vi "Packet RX Only.vi"() -> ()   [LabVIEW 2017, in "My Network Host v1.lvlib"]
uses:
  My Network Host v1.lvlib
  <vilib>/userdefined/Silver/nirio_resource_slv.ctl
  <vilib>/rvi/interface/common/niFpgaWaitOnOcc.vi
  <vilib>/Utility/error.llb/Error Cluster From Error Code.vi
  <vilib>/rvi/errors/niLvFpgaAdjustHostInterfaceError.vi
  <vilib>/FPGAPlugInAG/Dynamic/niLvFpga_Close_Dynamic.vi
  <vilib>/rvi/interface/nirviMethod/nirviMethod.xnode
  <vilib>/rvi/interface/nirviReadWriteControl/nirviReadWriteControl.xnode
  <vilib>/rvi/interface/nirviCloseFPGA/nirviCloseFPGA.xnode
  <vilib>/rvi/errors/niLvFpgaMergeErrorWithErrorCode.vi
  <vilib>/FPGAPlugInAG/Dynamic/niLvFpga_ConfigureFifo_Dynamic.vi
  <vilib>/FPGAPlugInAG/Dynamic/niLvFpga_StartFifo_Dynamic.vi
  NiFpgaLv.dll
  <vilib>/rvi/interface/Simulation/niFpgaSimulationCallBeginRW.vi
panel:
  out "size":i32
  out "data":u8[](array[numeric]) format="%.0x"
  out "byte enables":bool[](array[boolean])
  in  "resource name":T1="RIO0"
  in  "Local IP Address":string="169.254.122.140"
  out "string":string
  in  "UDP destination port":u16=12345
  out "MAC local address":u8[](array[numeric])=[0, 1, 2, 3, 4, 5] format="%.0x"
  in  "Promiscuous?":bool
  in  "Stop Button":bool
  out "data":u8[](array[numeric]) format="%.0x"
  # "Instructions\nNote: Compile the \"FPGA Top - Packet RX Only\" FPGA Target before running this VI. Error 7 \"File not found\" most likely means the bitfile has not been compiled yet.\n\n1. Configure \"Local IP Address\" for the IP you wish the FPGA to have\n2. Choose the UDP destination port that matches the configuration of the UDP transmitter\n3. Run the VI.\n4. Start a program to transmit packets to the Local IP Address/UDP destination port (the Simple UDP Sender example shipped with LabVIEW works well for this)."
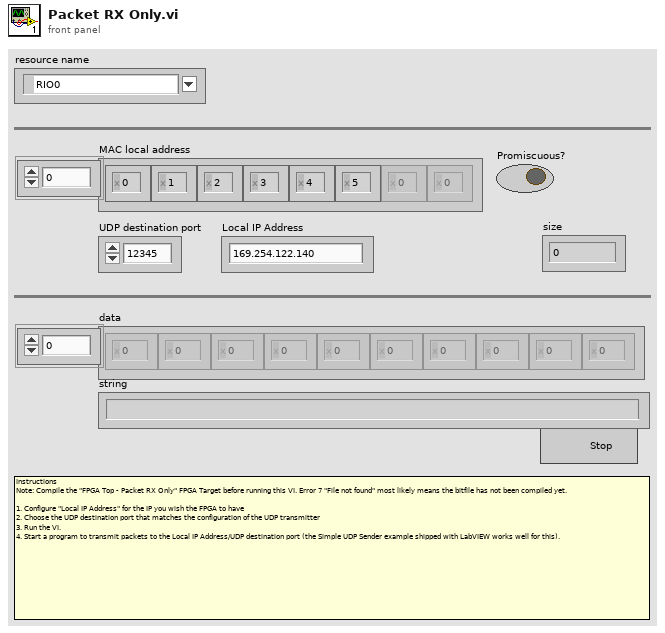
[diagram p1: front panel]
types:
  T1 = typedef "nirio_resource_slv.ctl" = tag
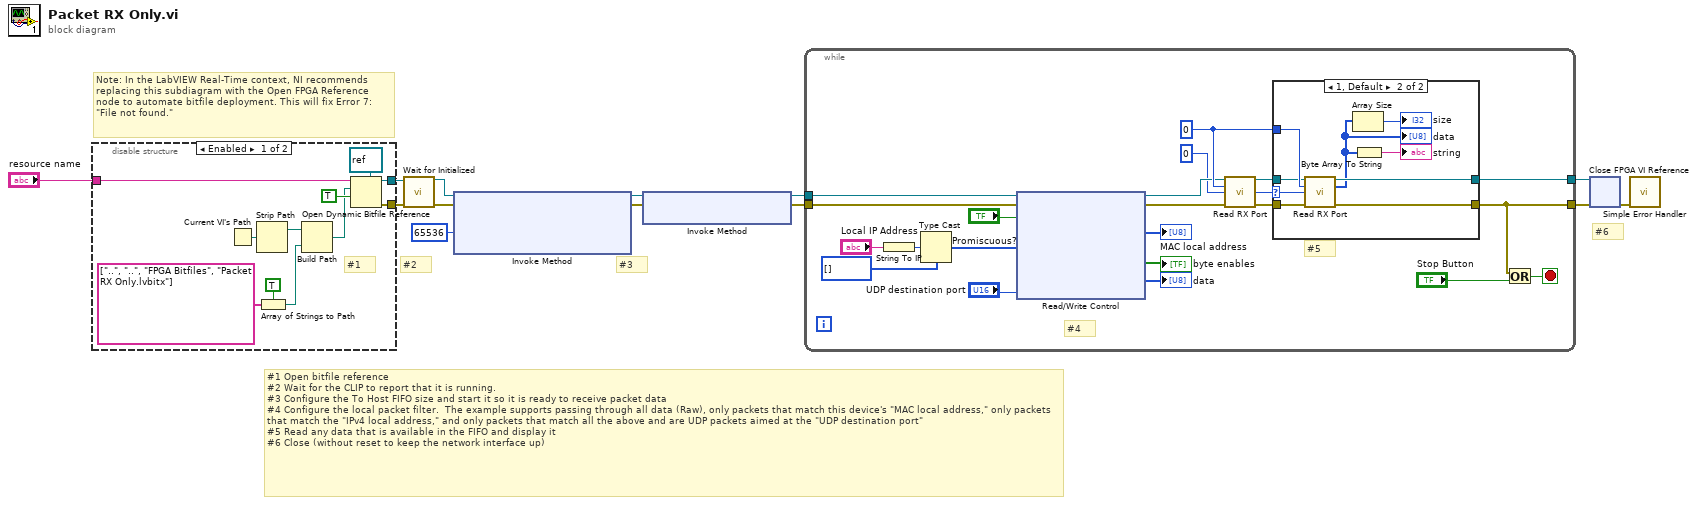
[diagram p0: block diagram]
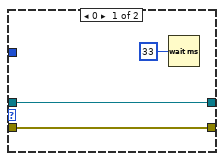
[diagram p3: hidden frame]
diagram:
  # "Note: In the LabVIEW Real-Time context, NI recommends replacing this subdiagram with the Open FPGA Reference node to automate bitfile deployment. This will fix Error 7: \"File not found.\""
  # "#6"
  # "#1 Open bitfile reference\n#2 Wait for the CLIP to report that it is running.\n#3 Configure the To Host FIFO size and start it so it is ready to receive packet data\n#4 Configure the local packet filter.  The example supports passing through all data (Raw), only packets that match this device's \"MAC local address,\" only packets that match the \"IPv4 local address,\" and only packets that match all the above and are UDP packets aimed at the \"UDP destination port\"\n#5 Read any data that is available in the FIFO and display it\n#6 Close (without reset to keep the network interface up)"
  # "#3"
  # "#2"
  n1 = disable-structure shown="Enabled" {
    disable-tunnel: "resource name" -> [w23 _]
    disable-tunnel: [w22 _] -> w2
    disable-tunnel: [w21 _] -> w1
    frame Enabled {
      # "#1"
      n2 = Current VI's Path() -> (path=w19:path)
      n3 = Strip Path(path=w19) -> (stripped path=w15:path)  [unwired: 1 out]
      n4 = Array of Strings to Path(0:string[] ["..", "..", "FPGA Bitfiles", "Packet RX Only.lvbitx"] ("array of strings"), 1:TRUE ("relative")) -> (2:w16:path)
      n5 = Build Path(base path=w15, name or relative path=w16) -> (appended path=w14:path)
      n6 = Open Dynamic Bitfile Reference(0:w23, 1:w14, 2:TRUE ("Run When Loaded"), 4:refnum<k20> refnum ("FPGA VI Reference Out")) -> (5:w22:refnum<k20>, 8:w21:errorcluster)  [unwired: 1 in]
    }
    frame Disabled {
      # "Insert code here for LabVIEW Real-Time"
    }
  }
  n7 = call "Wait for Initialized.vi"("Refnum in"=w2, "error in (no error)"=w1) -> ("Refnum out"=w4:refnum<k20>, "error out"=w5:errorcluster)  [unwired: 11 in, 1 out]
  n8 = xnode "Invoke Method"("FPGA VI Reference In"=w4, "error in"=w5, "Requested Depth"=u32 65536) -> ("FPGA VI Reference Out"=w10:refnum<k20>, "error out"=w7:errorcluster)  [unwired: 1 out]
  n9 = xnode "Invoke Method"("FPGA VI Reference In"=w10, "error in"=w7) -> ("FPGA VI Reference Out"=w8:refnum<k20>, "error out"=w6:errorcluster)
  n10 = while {
    tunnel: w8 -> [w29]
    tunnel: w6 -> [w37]
    tunnel: [w41] -> w13
    tunnel: [w40] -> w12
    stop <- w42 stop-if-true
    w46 = 0 ("Ethernet port")
    # "#5"
    # "#4"
    n11 = String To IP(1:"Local IP Address") -> (0:w31:u32)
    n12 = Type Cast(type=u8[] [] ("*(type *) &x"), x=w31) -> (*(type *) &x=w25:u8[])
    n13 = xnode "Read/Write Control"("FPGA VI Reference In"=w29, "error in"=w37, "Promiscuous?"="Promiscuous?", "IPv4 local address"=w25, "UDP destination port"="UDP destination port") -> ("FPGA VI Reference Out"=w38:refnum<k20>, "error out"=w36:errorcluster, "MAC local address"=→"MAC local address":u8[], "byte enables"=→"byte enables":bool[], "data"=→"data":u8[])
    n14 = call "Read RX Port.vi"("Refnum in"=w38, "Ethernet port"=w46, "Elements to Read"=u32 0, "error in (no error)"=w36) -> ("Refnum out"=w45:refnum<k20>, "Elements Remaining out"=w39:u32, "error out"=w44:errorcluster)  [unwired: 8 in, 1 out]
    n15 = case shown="1, Default" w39 {
      selector: w39 -> [_ w52]
      tunnel: w46 -> [_ w58]
      tunnel: w45 -> [w49 w57]
      tunnel: w44 -> [w48 w56]
      tunnel: [w48 w55] -> w41
      tunnel: [w49 w54] -> w40
      frame 0 {
        n16 = Wait (ms)(milliseconds to wait=u32 33) -> ()  [unwired: 1 out]
      }
      frame 1, Default {
        n17 = call "Read RX Port.vi"("Refnum in"=w57, "Ethernet port"=w58, "Elements to Read"=w52, "error in (no error)"=w56) -> ("Refnum out"=w54:refnum<k20>, "Data"=w51:u8[], "error out"=w55:errorcluster)  [unwired: 8 in, 1 out]
        "data" <- w51
        n18 = Array Size(array=w51) -> (size(s)=→"size":i32)
        n19 = Byte Array To String(unsigned byte array=w51) -> (string=→"string":string)
      }
    }
    n20 = Or(x=w41, y="Stop Button") -> (x .or. y?=w42:bool)
  }
  n21 = xnode "Close FPGA VI Reference"("FPGA VI Reference In"=w12, "error in"=w13) -> ("error out"=w11:errorcluster)
  n22 = call <vilib>:"Simple Error Handler.vi"("error in (no error)"=w11) -> ()  [unwired: 4 in, 5 out]
